vi "Module Not Stopped--error.vi"() -> (0 "error out":errorcluster)   [LabVIEW 2023, in "VoltageDataAquisition.lvlib"]
doc: "Outputs an error cluster containing a custom error code indicating the module was unable to synchronize the module finishing its clean up on exit.\n_____\nBased on DQMH Project Template 7.0.1.1316."
uses:
  VoltageDataAquisition.lvlib
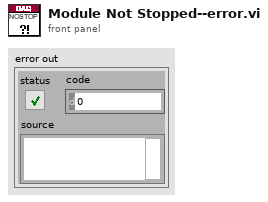
[diagram p1: front panel]
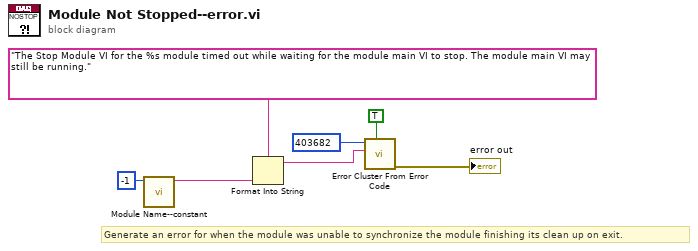
[diagram p0: block diagram]
diagram:
  # "Generate an error for when the module was unable to synchronize the module finishing its clean up on exit."
  n1 = call "Module Name--constant.vi"("Module ID"=-1) -> ("Module Name"=w2:string)  [unwired: 10 in]
  n2 = Format Into String(format string="The Stop Module VI for the %s module timed out while waiting for the module main VI to stop. The module main VI may still be running.", w2) -> (resulting string=w6:string)  [unwired: 2 in, 1 out]
  n3 = call <vilib>:"Error Cluster From Error Code.vi"("show call chain? (False)"=TRUE, "error message (\"\")"=w6, "error code (0)"=403682) -> ("error out"=→"error out":errorcluster)  [unwired: 6 in]
